vi "Error Cluster From Error Code.vi"(4 "is warning? (False)":bool, 6 "error in (no error)":errorcluster, 8 "error message (\"\")":string, 9 "error code (0)":i32) -> (0 "error out":errorcluster)   [LabVIEW 2019, in "Simple SysDef API.lvlib"]
doc: "Converts an error or warning code to an error cluster. This VI is useful when you receive a return value from a shared library call or when you return user-defined error codes."
uses:
  <userlib>/SimpleSysDef/Simple SysDef API.lvlib
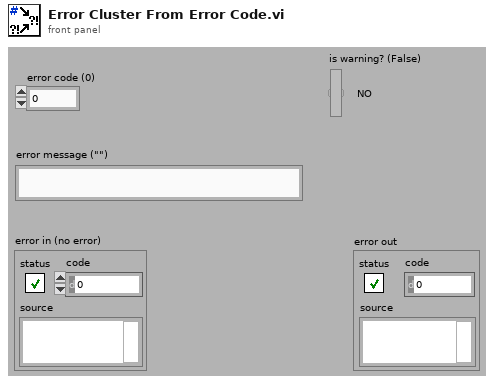
[diagram p1: front panel]
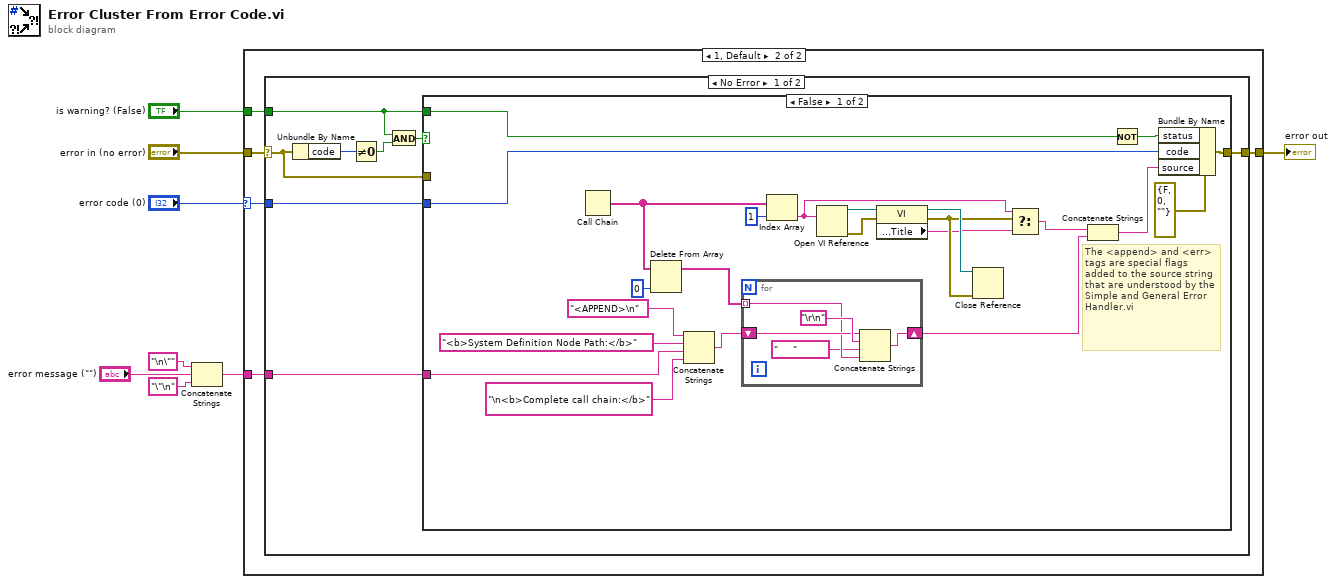
[diagram p0: block diagram]
diagram:
  n1 = Concatenate Strings("\n\"" ("source"), "error message (\"\")", "\"\n" ("source")) -> (w1:string)
  n2 = case shown="1, Default" "error code (0)" {
    selector: "error code (0)" -> [_ w12]
    tunnel: [w9 w14] -> w8
    tunnel: "error in (no error)" -> [w9 w13]
    tunnel: w1 -> [_ w11]
    tunnel: "is warning? (False)" -> [_ w10]
    frame 0 {
      # "If the error code in equals zero, then propagate the error in cluster regardless of its value."
    }
    frame 1, Default {
      n3 = case shown="No Error" w13 {
        selector: w13 -> [w17 w52]
        tunnel: [w22 w52] -> w14
        tunnel: w12 -> [w21 _]
        tunnel: w11 -> [w16 _]
        tunnel: w10 -> [w15 _]
        frame No Error {
          n4 = Unbundle By Name(w17) -> ("code"=w20:i32)
          n5 = Not Equal To 0?(x=w20) -> (x != 0?=w18:bool)
          n6 = And(x=w15, y=w18) -> (x .and. y?=w19:bool)
          n7 = case shown="False" w19 {
            tunnel: [w45 w51] -> w22
            tunnel: w21 -> [w41 _]
            tunnel: w17 -> [_ w51]
            tunnel: w15 -> [w31 _]
            tunnel: w16 -> [w23 _]
            frame False {
              # "The <append> and <err> tags are special flags added to the source string that are understood by the Simple and General Error Handler.vi"
              n8 = Call Chain() -> (call chain=w36:string[])
              n9 = Delete From Array(array=w36, index=0) -> (array with subset deleted=w29:string[])  [unwired: 1 in, 1 out]
              n10 = Concatenate Strings("<APPEND>\n", "<b>System Definition Node Path:</b>" ("call chain header"), w23, "\n<b>Complete call chain:</b>" ("call chain header")) -> (w27:string)
              n11 = for {
                tunnel: w29 -> [w47] mode=indexing
                shift-right: [w50] -> w25
                shift-left: w27 -> [w48]
                n12 = Concatenate Strings(w48, "\r\n", "     ", w47) -> (w50:string)
              }
              n13 = Index Array(array=w36, index=1) -> (element=w34:string)
              n14 = Open VI Reference(vi path=w34) -> (vi reference=w39:refnum<vi>, error out=w38:errorcluster)  [unwired: 5 in]
              n15 = property class="VI"(reference=w39, error in=w38) -> (reference out=w37:refnum<vi>, error out=w35:errorcluster, "Front Panel Window:Title"=w33:string)
              n16 = Close Reference(reference=w37, error in (no error)=w35) -> ()  [unwired: 1 out]
              n17 = Select(t=w34, s=w35, f=w33) -> (s? t:f=w32:string)
              n18 = Concatenate Strings(w32, w25) -> (w43:string)
              n19 = Not(x=w31) -> (.not. x?=w42:bool)
              n20 = Bundle By Name(cluster=errorcluster {"status"=FALSE, "code"=0, "source"=""} ("error out"), "status"=w42, "code"=w41, "source"=w43) -> (w45:errorcluster)
            }
            frame True {
              # "If the error code input is setting a warning, and a warning is already set on the wire, then we\ngo with the one already on the wire."
            }
          }
        }
        frame Error {
          # "An error in trumps any error code input."
        }
      }
    }
  }
  "error out" <- w8
